vi "Initialize MeasurementLink Session.vi"(7 "remote connection options":T2, 8 "error in (no error)":errorcluster, 9 "initialize and close session behavior":T1, 10 "session initialization parameters":T3, 11 "session factory in":refnum<class "Fake Session Factory.lvclass">) -> (0 "error out":errorcluster, 2 "session out":variant, 3 "session factory out":refnum<class "Fake Session Factory.lvclass">)   [LabVIEW 2020, in "MeasurementServerTests.lvlib" / "Fake Session Factory.lvclass"]
uses:
  Fake Session Factory.lvclass
  Runtime/MeasurementLink Instrument/ISession Factory/Session Initialization Parameters.ctl
  Runtime/MeasurementLink Instrument/ISession Factory/Remote Connection Options.ctl
  Runtime/MeasurementLink Instrument/ISession Factory/Initialize and Close Session Behavior.ctl
  Call Recorder Action.ctl
  Runtime/MeasurementLink Instrument/ISession Factory/ISession Factory.lvclass
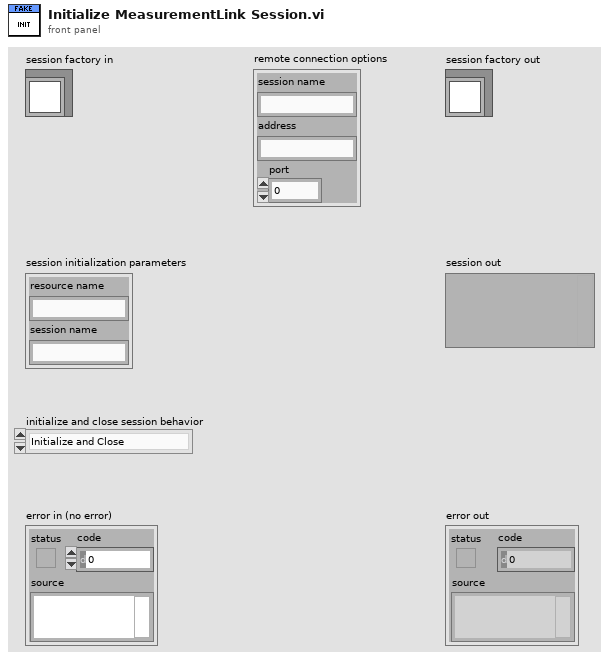
[diagram p1: front panel]
types:
  T1 = typedef "MeasurementLink Instrument.lvlib/ISession Factory.lvclass/Initialize and Close Session Behavior.ctl" = enum16{"Initialize and Close", "Attach and Detach", "Initialize and Detach", "Attach and Close"}
  T2 = typedef "MeasurementLink Instrument.lvlib/ISession Factory.lvclass/Remote Connection Options.ctl" = cluster{"session name":string, "address":string, "port":u32}
  T3 = typedef "MeasurementLink Instrument.lvlib/ISession Factory.lvclass/Session Initialization Parameters.ctl" = cluster{"resource name":string, "session name":string}
  T4 = typedef "MeasurementServerTests.lvlib/Fake Session Factory.lvclass/Call Recorder Action.ctl" = enum16{"Initialize", "Read Values", "Record Initialize-Initialize", "Record Initialize-Attach", "Record Close-Close", "Record Close-Detach"}
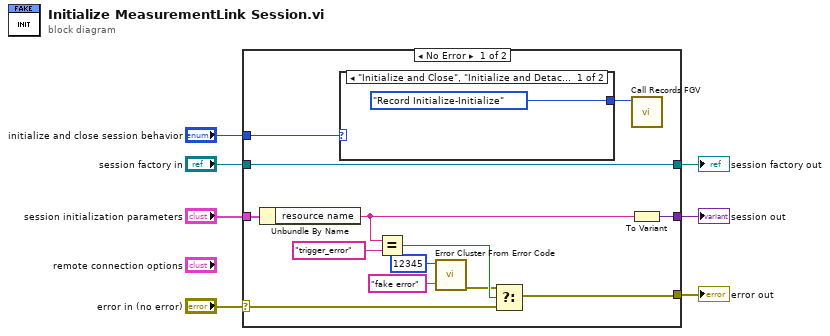
[diagram p0: block diagram]
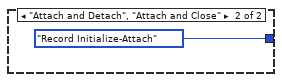
[diagram p2: hidden frame]
diagram:
  n1 = case shown="No Error" "error in (no error)" {
    selector: "error in (no error)" -> [w10 w24]
    tunnel: "session initialization parameters" -> [w16 _]
    tunnel: [w20 _] -> w6
    tunnel: [w12 w24] -> w4
    tunnel: "session factory in" -> [w19 w23]
    tunnel: [w19 w23] -> w2
    tunnel: "initialize and close session behavior" -> [w18 _]
    frame No Error {
      n2 = Unbundle By Name(w16) -> ("resource name"=w8:string)
      n3 = case shown="\"Initialize and Close\", \"Initialize and Detach\"" w18 {
        tunnel: [Call_Recorder_Action."Record Initialize-Initialize" ("Call Recorder Action") Call_Recorder_Action."Record Initialize-Attach" ("Call Recorder Action")] -> w17
        frame "Initialize and Close", "Initialize and Detach" {
        }
        frame "Attach and Detach", "Attach and Close" {
        }
      }
      n4 = Equal?(x=w8, y="trigger_error") -> (x = y?=w11:bool)
      n5 = call <vilib>:"Error Cluster From Error Code.vi"("error message (\"\")"="fake error" ("error message (\"\")"), "error code (0)"=12345) -> ("error out"=w9:errorcluster)  [unwired: 7 in]
      n6 = Select(t=w9, s=w11, f=w10) -> (s? t:f=w12:errorcluster)
      n7 = call "Call Records FGV.vi"("Call Recorder Action"=w17) -> ()  [unwired: 7 in, 4 out]
      n8 = To Variant(anything=w8) -> (Variant=w20:variant)
    }
    frame Error {
    }
  }
  "error out" <- w4
  "session factory out" <- w2
  "session out" <- w6
